vi "oldMyHostCode.vi"() -> ()   [LabVIEW 2013, in "MyHostCode.lvlib"]
doc: "This VI was generated automatically using the FPGA Wizard. You can modify the VI normally."
uses:
  MyHostCode.lvlib
  FPGACode/Lead Enum.ctl
  Trigger Params.ctl
  <vilib>/rvi/interface/common/niFpgaWaitOnOcc.vi
  <vilib>/FPGAPlugInAG/USB-7856R/niLvFpga_Open_USB-7856R.vi
  <vilib>/rvi/interface/common/dynamic/niFpgaDynamicAddResources.vi
  <vilib>/FPGAPlugInAG/Dynamic/niLvFpga_Reset_Dynamic.vi
  <vilib>/FPGAPlugInAG/Dynamic/niLvFpga_Run_Dynamic.vi
  <vilib>/Utility/error.llb/Error Cluster From Error Code.vi
  <vilib>/rvi/errors/niLvFpgaAdjustHostInterfaceError.vi
  <vilib>/Utility/file.llb/Write To Spreadsheet File (I64).vi
  <vilib>/FPGAPlugInAG/Dynamic/niLvFpga_Close_Dynamic.vi
  <vilib>/rvi/interface/nirviOpenFPGA/nirviOpenFPGA.xnode
  FPGA Bitfiles/ECGPWMAdaptiveFi_FPGATarget2_ECGAFSPIInput_rwhZEZktnWM.lvbitx
  <vilib>/rvi/interface/nirviMethod/nirviMethod.xnode
  <vilib>/rvi/interface/nirviReadWriteControl/nirviReadWriteControl.xnode
  <vilib>/rvi/interface/nirviCloseFPGA/nirviCloseFPGA.xnode
  <vilib>/rvi/interface/Simulation/niFpgaSimulationCallBeginRW.vi
  <vilib>/FPGAPlugInAG/Dynamic/niLvFpga_ReadFifo_Dynamic.vi
  <vilib>/rvi/errors/niLvFpgaMergeErrorWithErrorCode.vi
  NiFpgaLv.dll
panel:
  out "Waveform Chart":i16[](graph)
  out "Trigger":i16[](graph)
  in  "Trigger":T1={"Channel"=enum."II", "Threshold"=1000, "Invert"=FALSE}
  in  "High Pass":bool
  out "Loop Time":u32
  in  "Reset":bool
  out "Waveform Graph":dbl[](graph)
  out "Waveform Graph 2":dbl[](graph)
  out "WeightSum":fxp<+/-,33,19> format="%.20g"
  out "BetaProduct":fxp<+/-,32,-1> format="%.33g"
  in  "Filter Size":i16=100
  out "Invasive Blood Pressure":i16[][](graph)
  in  "Plot Info":T3={"Element"={"Lead"=enum."RA", "Filter"=FALSE}, "Element 2"={"Lead"=enum."RA", "Filter"=TRUE}, "Element 3"={"Lead"=enum."LA", "Filter"=FALSE}, "Element 4"={"Lead"=enum."LA", "Filter"=TRUE}, "Element 5"={"Lead"=enum."LL", "Filter"=FALSE}, "Element 6"={"Lead"=enum."LL", "Filter"=TRUE}, "Element 7"={"Lead"=enum."II", "Filter"=TRUE}, "Element 8"={"Lead"=enum."III", "Filter"=TRUE}}
  in  "file path (dialog if empty)":path
  in  "Record":bool
  out "Gradients":i16[][](graph)
  in  "Filter On":bool=TRUE
  out "ECG":i16[][](graph)
  out "Actual Loop Rate (Ticks)":u32
  in  "Beta":fxp<+/-,32,-16>
  out "Late? Latched":bool
  in  "Start 0":bool
  in  "Loop Rate (Hz)":dbl=10000.0
  out "Calculated Rate (Hz)":dbl
  out "error out":errorcluster
  in  "Global Stop":bool
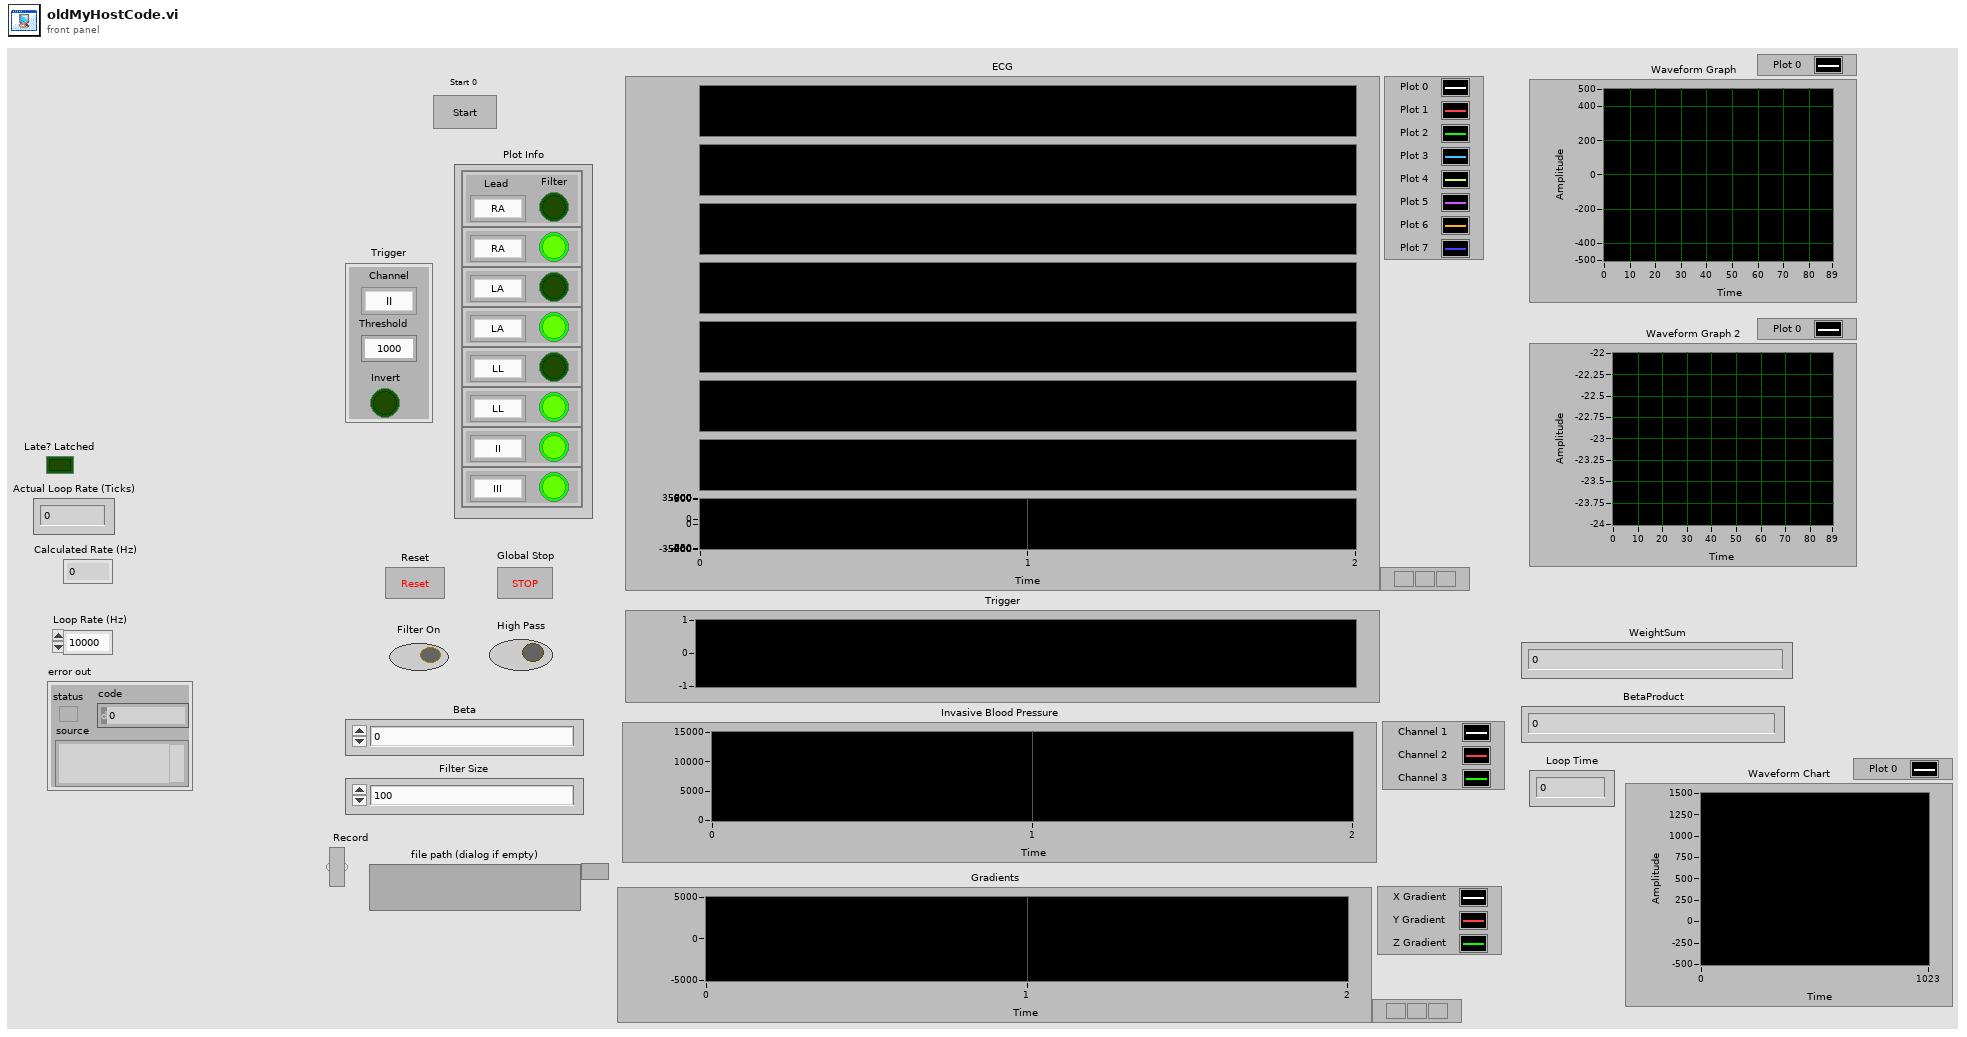
[diagram p1: front panel]
types:
  T1 = typedef "Trigger Params.ctl" = cluster{"Channel":T2, "Threshold":i16, "Invert":bool}
  T2 = typedef "Lead Enum.ctl" = enum16{"RA", "LA", "LL", "V1", "V2", "V3", "V4", "V5", "V6", "I", "II", "III", "aVR", "aVL", "aVF", "Vw"}
  T3 = cluster{"Element":cluster{"Lead":T2, "Filter":bool}, "Element 2":cluster{"Lead":T2, "Filter":bool}, "Element 3":cluster{"Lead":T2, "Filter":bool}, "Element 4":cluster{"Lead":T2, "Filter":bool}, "Element 5":cluster{"Lead":T2, "Filter":bool}, "Element 6":cluster{"Lead":T2, "Filter":bool}, "Element 7":cluster{"Lead":T2, "Filter":bool}, "Element 8":cluster{"Lead":T2, "Filter":bool}}
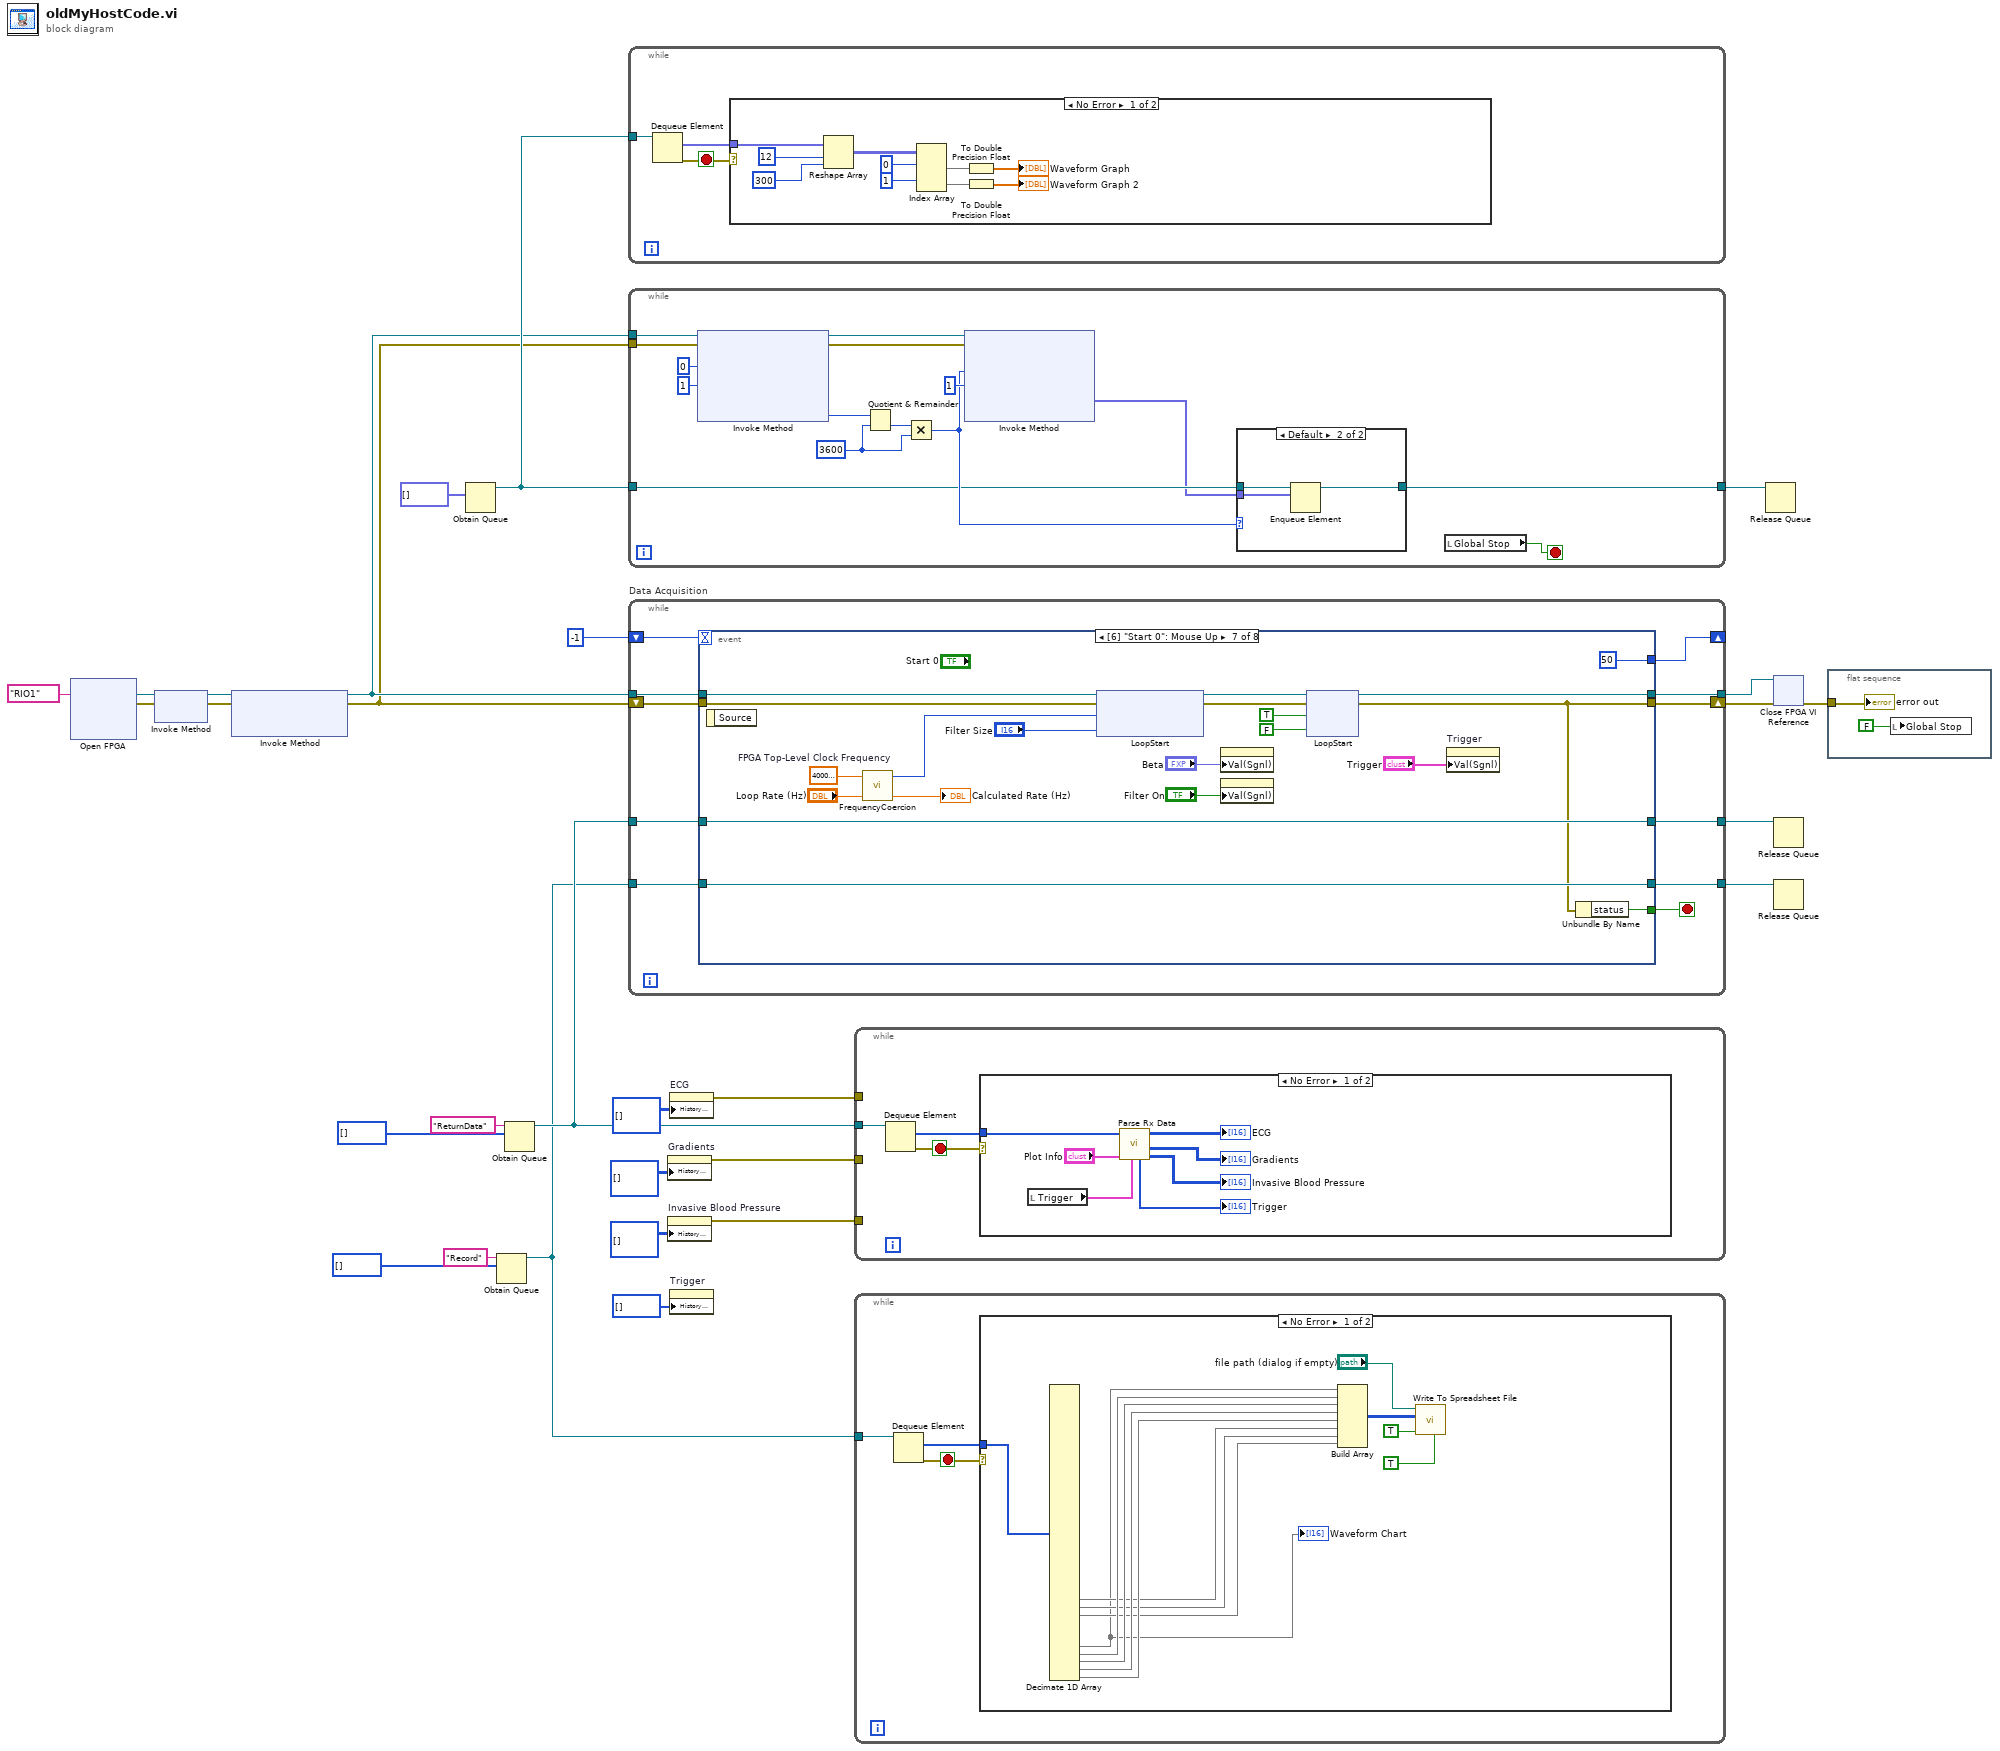
[diagram p0: block diagram]
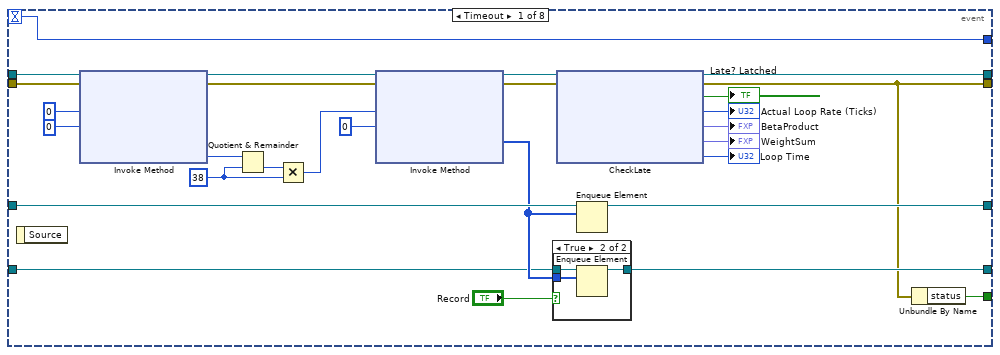
[diagram p2: hidden frame]
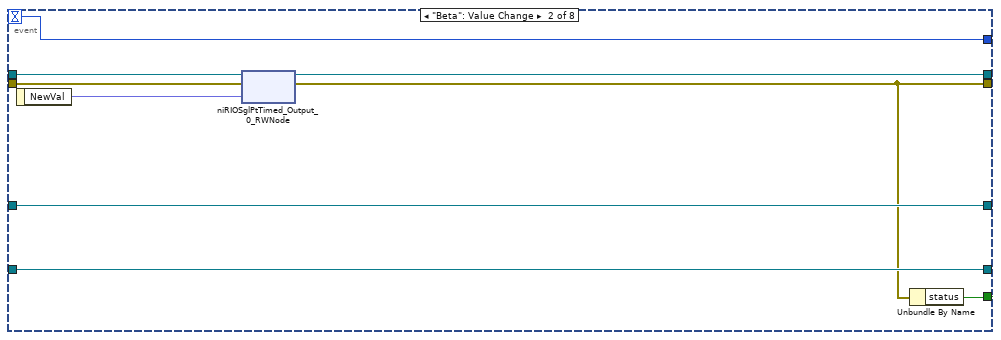
[diagram p4: hidden frame]
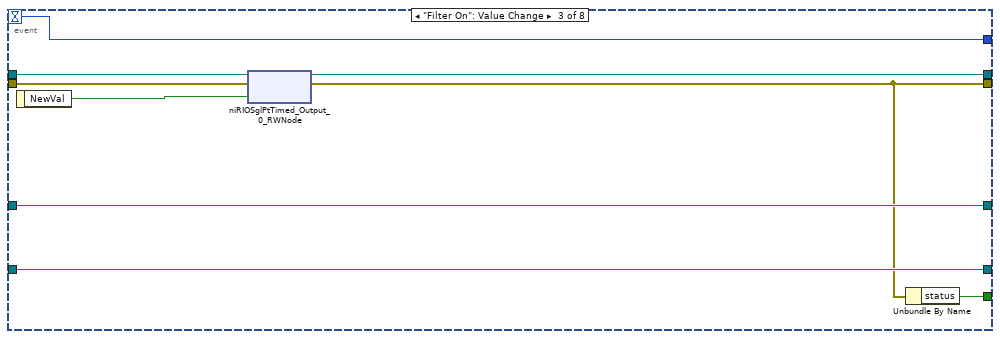
[diagram p5: hidden frame]
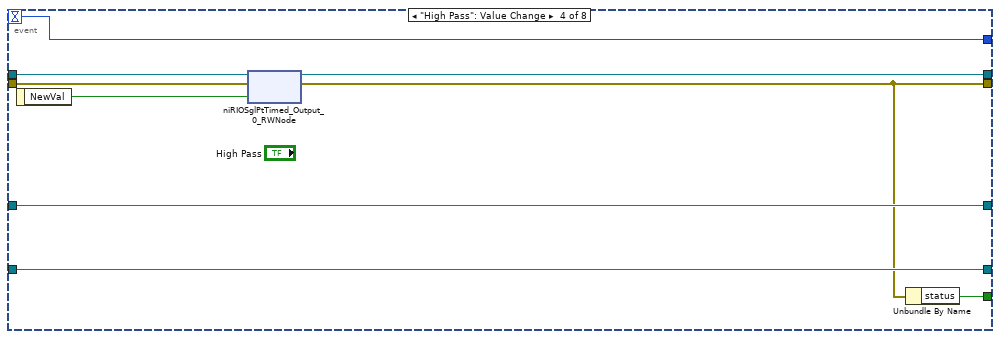
[diagram p6: hidden frame]
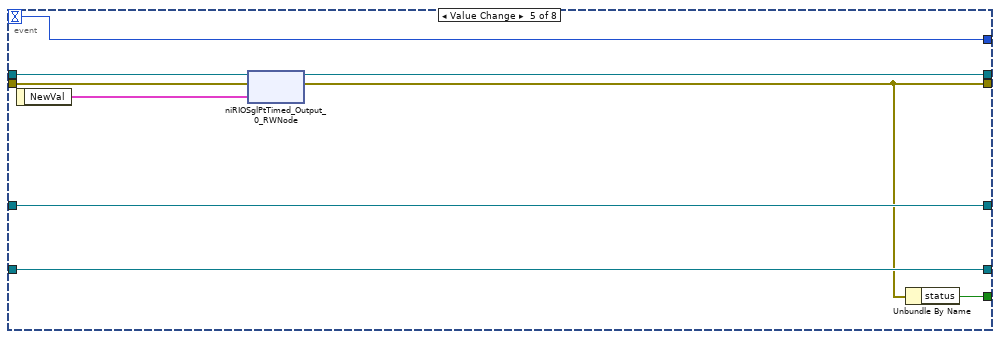
[diagram p7: hidden frame]
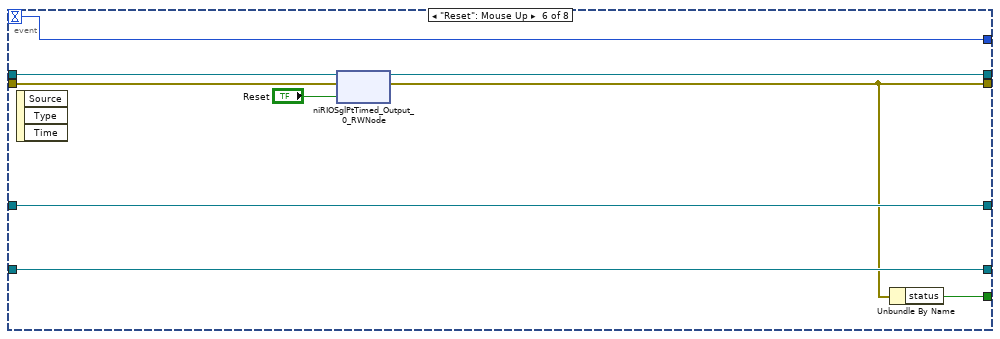
[diagram p8: hidden frame]
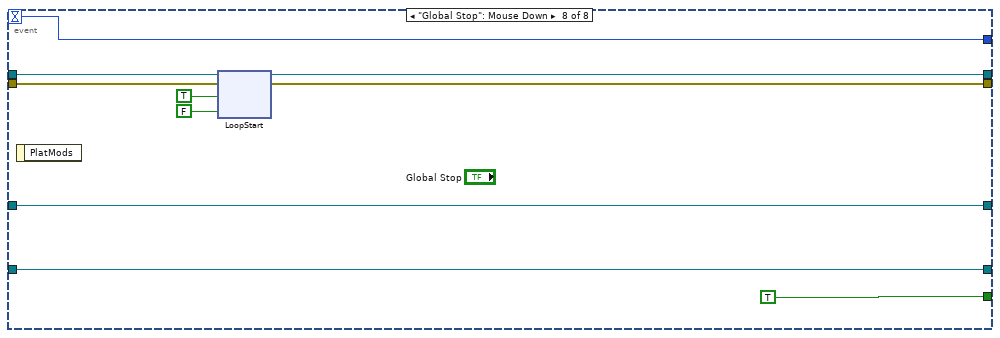
[diagram p9: hidden frame]
diagram:
  n1 = xnode ("Open FPGA")("resource name"=tag "RIO1") -> ("FPGA VI Reference Out"=w28:refnum<k20>, "error out"=w27:errorcluster)  [unwired: 1 in]
  n2 = xnode ("Invoke Method")("FPGA VI Reference In"=w28, "error in"=w27) -> ("FPGA VI Reference Out"=w5:refnum<k20>, "error out"=w29:errorcluster)
  n3 = xnode ("Invoke Method")("FPGA VI Reference In"=w5, "error in"=w29) -> ("FPGA VI Reference Out"=w3:refnum<k20>, "error out"=w2:errorcluster)  [unwired: 1 in]
  n4 = Obtain Queue(element data type=fxp<+/-,32,16>[] [] ("Data")) -> (queue out=w8:refnum<queue>)  [unwired: 4 in, 2 out]
  n5 = Obtain Queue(name (unnamed)="Record", element data type=i16[] []) -> (queue out=w13:refnum<queue>)  [unwired: 3 in, 2 out]
  n6 = Obtain Queue(name (unnamed)="ReturnData", element data type=i16[] []) -> (queue out=w21:refnum<queue>)  [unwired: 3 in, 2 out]
  n7 = while {
    tunnel: w8 -> [w32]
    stop <- w30 stop-if-true
    n8 = Dequeue Element(queue=w32) -> (element=w31:fxp<+/-,32,16>[], error out=w30:errorcluster)  [unwired: 2 in, 2 out]
    n9 = case shown="No Error" w30 {
      tunnel: w31 -> [w42 _]
      frame No Error {
        n10 = Reshape Array(w42, 12 ("dimension size"), 300 ("dimension size")) -> (w38:fxp<+/-,32,16>[][])
        n11 = Index Array(array=w38, index (row) #1=0 ("index (row)"), index (row) #2=1 ("index (row)")) -> (element #1=w37:fxp<+/-,32,16>[], element #2=w35:fxp<+/-,32,16>[])  [unwired: 2 in]
        n12 = To Double Precision Float(number=w37) -> (double precision float=→"Waveform Graph":dbl[])
        n13 = To Double Precision Float(number=w35) -> (double precision float=→"Waveform Graph 2":dbl[])
      }
      frame Error {
      }
    }
  }
  n14 = while {
    tunnel: w3 -> [w57]
    tunnel: w2 -> [w56]
    tunnel: w8 -> [w45]
    tunnel: [w43] -> w7
    stop <- w48 stop-if-true
    w50 = u32 3600 ("y")
    n15 = xnode "Invoke Method"("FPGA VI Reference In"=w57, "error in"=w56, "Number of Elements"=u32 0, "Timeout (ms)"=1) -> ("FPGA VI Reference Out"=w53:refnum<k20>, "error out"=w52:errorcluster, "Elements Remaining"=w49:u32)  [unwired: 1 out]
    n16 = Quotient & Remainder(x=w49, y=w50) -> (floor(x/y)=w51:u32)  [unwired: 1 out]
    n17 = Multiply(x=w51, y=w50) -> (x*y=w46:u32)
    n18 = xnode "Invoke Method"("FPGA VI Reference In"=w53, "error in"=w52, "Number of Elements"=w46, "Timeout (ms)"=1) -> ("Data"=w44:fxp<+/-,32,16>[])  [unwired: 3 out]
    n19 = case shown="Default" w46 {
      tunnel: w45 -> [w58 w61]
      tunnel: w44 -> [_ w60]
      tunnel: [w58 w59] -> w43
      frame 0 {
      }
      frame Default {
        n20 = Enqueue Element(queue=w61, element=w60) -> (queue out=w59:refnum<queue>)  [unwired: 2 in, 2 out]
      }
    }
    n21 = local read "Global Stop"() -> (w48:bool)
  }
  n22 = while "Data Acquisition" {
    tunnel: w3 -> [w68]
    shift-right: [w72] -> w26
    shift-left: w2 -> [w69]
    tunnel: [w70] -> w24
    tunnel: w21 -> [w67]
    tunnel: [w66] -> w16
    tunnel: w13 -> [w65]
    tunnel: [w64] -> w12
    shift-right: [w62] -> _
    shift-left: -1 -> [w63]
    stop <- w71 stop-if-true
    n23 = event shown="[6] \"Start 0\": Mouse Up" {
      selector: _ -> [_ _ _ _ _ _ _ _]
      dyn-events: _ -> [_ _ _ _ _ _ _ _]
      timeout: w63 -> [w75 w107 w116 w125 w134 w143 _ w172]
      tunnel: [w74 w106 w115 w124 w133 w142 w152 w173] -> w72
      tunnel: [w73 w105 w114 w123 w132 w141 w151 TRUE] -> w71
      tunnel: [w100 w111 w120 w129 w138 w147 w157 w174] -> w70
      tunnel: w69 -> [w77 w112 w121 w130 w139 w148 w167 w175]
      tunnel: w68 -> [w78 w113 w122 w131 w140 w149 w168 w176]
      tunnel: w67 -> [w89 w109 w118 w127 w136 w146 w166 w179]
      tunnel: [w85 w109 w118 w127 w136 w146 w166 w179] -> w66
      tunnel: w65 -> [w82 w108 w117 w126 w135 w145 w165 w178]
      tunnel: [w76 w108 w117 w126 w135 w145 w165 w178] -> w64
      tunnel: [w75 w107 w116 w125 w134 w143 50 w172] -> w62
      event Timeout {
        w87 = u32 38 ("y")
        n24 = event-data() -> ()  [unwired: 1 in, 1 out]
        n25 = xnode "Invoke Method"("FPGA VI Reference In"=w78, "error in"=w77, "Number of Elements"=u32 0, "Timeout (ms)"=0) -> ("FPGA VI Reference Out"=w95:refnum<k20>, "error out"=w94:errorcluster, "Elements Remaining"=w93:u32)  [unwired: 1 out]
        n26 = Quotient & Remainder(x=w93, y=w87) -> (floor(x/y)=w88:u32)  [unwired: 1 out]
        n27 = Multiply(x=w88, y=w87) -> (x*y=w86:u32)
        n28 = xnode "Invoke Method"("FPGA VI Reference In"=w95, "error in"=w94, "Number of Elements"=w86, "Timeout (ms)"=0) -> ("FPGA VI Reference Out"=w91:refnum<k20>, "error out"=w90:errorcluster, "Data"=w83:i16[])  [unwired: 1 out]
        n29 = case shown="True" "Record" {
          tunnel: w83 -> [_ w104]
          tunnel: w82 -> [w101 w103]
          tunnel: [w101 w102] -> w76
          frame False {
          }
          frame True {
            n30 = Enqueue Element(queue=w103, element=w104) -> (queue out=w102:refnum<queue>)  [unwired: 2 in, 2 out]
          }
        }
        n31 = xnode ("CheckLate")("FPGA VI Reference In"=w91, "error in"=w90) -> ("FPGA VI Reference Out"=w100:refnum<k20>, "error out"=w74:errorcluster, "Late? Latched"=→"Late? Latched":bool, "Actual Loop Rate (Ticks)"=→"Actual Loop Rate (Ticks)":u32, "BetaProduct"=→"BetaProduct":fxp<+/-,32,-1>, "WeightSum"=→"WeightSum":fxp<+/-,33,19>, "Loop Time"=→"Loop Time":u32)
        n32 = Enqueue Element(queue=w89, element=w83) -> (queue out=w85:refnum<queue>)  [unwired: 2 in, 2 out]
        n33 = Unbundle By Name(w74) -> ("status"=w73:bool)
      }
      event "Beta": Value Change {
        n34 = event-data() -> ("NewVal"=w110:fxp<+/-,32,-16>)  [unwired: 1 in]
        n35 = xnode ("niRIOSglPtTimed_Output_0_RWNode")("FPGA VI Reference In"=w113, "error in"=w112, "Beta"=w110) -> ("FPGA VI Reference Out"=w111:refnum<k20>, "error out"=w106:errorcluster)
        n36 = Unbundle By Name(w106) -> ("status"=w105:bool)
      }
      event "Filter On": Value Change {
        n37 = event-data() -> ("NewVal"=w119:bool)  [unwired: 1 in]
        n38 = xnode ("niRIOSglPtTimed_Output_0_RWNode")("FPGA VI Reference In"=w122, "error in"=w121, "Filter On"=w119) -> ("FPGA VI Reference Out"=w120:refnum<k20>, "error out"=w115:errorcluster)
        n39 = Unbundle By Name(w115) -> ("status"=w114:bool)
      }
      event "High Pass": Value Change {
        n40 = event-data() -> ("NewVal"=w128:bool)  [unwired: 1 in]
        n41 = xnode ("niRIOSglPtTimed_Output_0_RWNode")("FPGA VI Reference In"=w131, "error in"=w130, "HPF"=w128) -> ("FPGA VI Reference Out"=w129:refnum<k20>, "error out"=w124:errorcluster)
        n42 = Unbundle By Name(w124) -> ("status"=w123:bool)
      }
      event Value Change {
        n43 = event-data() -> ("NewVal"=w137:T1)  [unwired: 1 in]
        n44 = xnode ("niRIOSglPtTimed_Output_0_RWNode")("FPGA VI Reference In"=w140, "error in"=w139, "Trigger"=w137) -> ("FPGA VI Reference Out"=w138:refnum<k20>, "error out"=w133:errorcluster)
        n45 = Unbundle By Name(w133) -> ("status"=w132:bool)
      }
      event "Reset": Mouse Up {
        n46 = event-data() -> ()  [unwired: 1 in, 3 out]
        n47 = xnode ("niRIOSglPtTimed_Output_0_RWNode")("FPGA VI Reference In"=w149, "error in"=w148, "Reset"="Reset") -> ("FPGA VI Reference Out"=w147:refnum<k20>, "error out"=w142:errorcluster)
        n48 = Unbundle By Name(w142) -> ("status"=w141:bool)
      }
      event "Start 0": Mouse Up {
        w164 = 40000000.0  # FPGA Top-Level Clock Frequency
        n49 = event-data() -> ()  [unwired: 1 in, 1 out]
        n50 = call "FrequencyCoercion.vi"("Loop Rate (Hz)"="Loop Rate (Hz)", "FPGA Top-Level Clock Frequency"=w164) -> ("Actual Rate (Hz)"=→"Calculated Rate (Hz)":dbl, "FPGA Ticks"=w161:u32)  [unwired: 2 in]
        n51 = xnode ("LoopStart")("FPGA VI Reference In"=w168, "error in"=w167, "Loop Rate (Ticks)"=w161, "Filter Size"="Filter Size") -> ("FPGA VI Reference Out"=w159:refnum<k20>, "error out"=w158:errorcluster)
        n52 = property on="Beta" class="DigNum (strict)"("Val(Sgnl)"="Beta") -> ()  [unwired: 2 in, 2 out]
        n53 = property on="Filter On" class="Bool (strict)"("Val(Sgnl)"="Filter On") -> ()  [unwired: 2 in, 2 out]
        n54 = xnode ("LoopStart")("FPGA VI Reference In"=w159, "error in"=w158, "Start 0"=TRUE, "Start 0"=FALSE) -> ("FPGA VI Reference Out"=w157:refnum<k20>, "error out"=w152:errorcluster)
        n55 = property on="Trigger" class="Clust (strict)"("Val(Sgnl)"="Trigger") -> ()  [unwired: 2 in, 2 out]
        n56 = Unbundle By Name(w152) -> ("status"=w151:bool)
      }
      event "Global Stop": Mouse Down {
        n57 = event-data() -> ()  [unwired: 1 in, 1 out]
        n58 = xnode ("LoopStart")("FPGA VI Reference In"=w176, "error in"=w175, "stop"=TRUE, "stop"=FALSE) -> ("FPGA VI Reference Out"=w174:refnum<k20>, "error out"=w173:errorcluster)
      }
    }
  }
  n59 = property on="Gradients" class="WFChart (strict)"("History Data"=i16[][] []) -> (error out=w18:errorcluster)  [unwired: 2 in, 1 out]
  n60 = property on="Invasive Blood Pressure" class="WFChart (strict)"("History Data"=i16[][] []) -> (error out=w10:errorcluster)  [unwired: 2 in, 1 out]
  n61 = property on="ECG" class="WFChart (strict)"("History Data"=i16[][] []) -> (error out=w19:errorcluster)  [unwired: 2 in, 1 out]
  n62 = property on="Trigger" class="WFChart (strict)"("History Data"=i16[] []) -> ()  [unwired: 2 in, 2 out]
  n63 = while {
    tunnel: w21 -> [w182]
    tunnel: w19 -> [_]
    tunnel: w18 -> [_]
    tunnel: w10 -> [_]
    stop <- w181 stop-if-true
    n64 = Dequeue Element(queue=w182) -> (element=w180:i16[], error out=w181:errorcluster)  [unwired: 2 in, 2 out]
    n65 = case shown="No Error" w181 {
      tunnel: w180 -> [w188 _]
      frame No Error {
        n66 = local read "Trigger"() -> (w184:T1)
        n67 = call "Parse Rx Data.vi"("Trigger"=w184, "Plot Info"="Plot Info", "Input Data"=w188) -> ("Pressures"=→"Invasive Blood Pressure":i16[][], "Gradients"=→"Gradients":i16[][], "ECG Data"=→"ECG":i16[][], "Trigger"=→"Trigger":i16[])  [unwired: 5 in]
      }
      frame Error {
      }
    }
  }
  n68 = while {
    tunnel: w13 -> [w190]
    stop <- w192 stop-if-true
    n69 = Dequeue Element(queue=w190) -> (element=w191:i16[], error out=w192:errorcluster)  [unwired: 2 in, 2 out]
    n70 = case shown="No Error" w192 {
      tunnel: w191 -> [w202 _]
      frame No Error {
        n71 = Decimate 1D Array(w202) -> (w195:i16[], w196:i16[], w197:i16[], w193:i16[], w201:i16[], w200:i16[], w199:i16[], w198:i16[])  [unwired: 30 out]
        "Waveform Chart" <- w193
        n72 = Build Array(w193, w201, w200, w199, w198, w195, w196, w197) -> (w194:i16[][])
        n73 = call-poly <vilib>:"Write To Spreadsheet File.vi"("transpose? (no:F)"=TRUE, "append to file? (new file:F)"=TRUE, "2D data"=w194, "file path (dialog if empty)"="file path (dialog if empty)") -> ()  [unwired: 4 in, 1 out]
      }
      frame Error {
      }
    }
  }
  n74 = Release Queue(queue=w7) -> ()  [unwired: 2 in, 3 out]
  n75 = xnode ("Close FPGA VI Reference")("FPGA VI Reference In"=w24, "error in"=w26) -> ("error out"=w25:errorcluster)
  n76 = Release Queue(queue=w16) -> ()  [unwired: 2 in, 3 out]
  n77 = Release Queue(queue=w12) -> ()  [unwired: 2 in, 3 out]
  n78 = flat-sequence {
    tunnel: w25 -> [w207]
    frame #0 {
      n79 = local write "Global Stop"(FALSE ("Global Stop")) -> ()
      "error out" <- w207
    }
  }
